vi "FT10_Fornax Energy Parameter Command.vi"(0 "Energy Channel ID":T4, 1 "Generator":T6="{\"Partition\":\"", 5 "Instrument Type":T5, 7 "Parameter Type":T3, 9 "Parameter Value":T2, 11 "Energy Mode":T1) -> (4 "JSON Command":string)   [LabVIEW 2015]
doc: "Build JSON command to adjust the mode or power on a specific port via Fornax. See Fornax manual > \"EnergyParameterCommand\" for more details."
uses:
  Controls/Control_Fornax Generator.ctl
  Controls/Control_Fornax Instrument Type.ctl
  Controls/Control_Fornax Energy Channel ID.ctl
  Controls/Control_Fornax Parameter Type.ctl
  Controls/Control_Fornax Parameter Value.ctl
  Controls/Control_Fornax Energy Mode.ctl
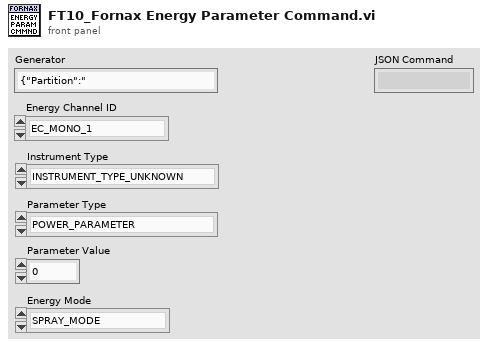
[diagram p1: front panel]
types:
  T1 = typedef "Control_Fornax Energy Mode.ctl" = enum16{"SPRAY_MODE", "CUT_MODE", "BLEND_MODE", "FULGERATE_MODE", "BIPOLAR_MODE", "VESSEL_SEALING_MODE", "VALLEYLAB_MODE", "BIPOLAR_RESECTION_CUT_MODE", "BIPOLAR_RESECTION_COAG_MODE", "AUTOBIPOLAR_MODE", "VIPER_HLA", "SOFT_COAG_MODE", "ECUT_MODE", "SHARED_SPRAY_MODE", "SHARED_FULGERATE_MODE", "CARDIO_MONO_MODE", "CARDIO_BIPOLAR_MODE", "BIPOLAR_LOW_MODE", "BIPOLAR_MACRO_MODE", "BIPOLAR_STANDARD_MODE", "BIPOLAR_MEDIUM_MODE", "VL_ENDOSCOPY_MODE", "NUM_ENERGY_MODES"}
  T2 = typedef "Control_Fornax Parameter Value.ctl" = i32
  T3 = typedef "Control_Fornax Parameter Type.ctl" = enum16{"POWER_PARAMETER", "CUT_MODALITY_POWER_PARAMETER", "COAG_MODALITY_POWER_PARAMETER", "VL_MODALITY_POWER_PARAMETER", "BY_MODE_POWER_PARAMETER", "VL_ENDO_CUT_MODALITY_POWER_PARAMETER", "VL_ENDO_COAG_MODALITY_POWER_PARAMETER", "VL_ENDO_COAG_ON_CUT_MODALITY_POWER_PARAMETER", "MODE_PARAMETER   (for changing Bipolar mode)", "CUT_MODALITY_MODE_PARAMETER  (for changing monopolar cut mode)", "COAG_MODALITY_MODE_PARAMETER (for changing monopolar coag mode)", "VL_ENDO_COAG_MODALITY_MODE_PARAMETER", "VL_ENDO_CUT_INTERVAL_PARAMETER", "VL_ENDO_CUT_DURATION_PARAMETER", "POWER_BAR_PARAMETER", "MAX_ACTIVATION_MSEC_TIME_PARAMETER", "AUTOBIPOLAR_DELAY_MSEC_TIME", "VL_ENDO_COAG_QUICK_ACCESS_PARAMETER"}
  T4 = typedef "Control_Fornax Energy Channel ID.ctl" = enum16{"EC_MONO_1  ", "EC_BIPOLAR  ", "EC_MONO_2  ", "EC_ADVANCED  ", "EC_ADVANCED_ECUT  ", "EC_ADVANCED_DCUT  ", "EC_SHARED_COAG  ", "EC_INTERNAL_BIP_CAL  "}
  T5 = typedef "Control_Fornax Instrument Type.ctl" = enum16{"INSTRUMENT_TYPE_UNKNOWN", "INSTRUMENT_TYPE_MONOPOLAR", "INSTRUMENT_TYPE_BIPOLAR", "INSTRUMENT_TYPE_TRIVERSE", "INSTRUMENT_TYPE_LIGASURE", "INSTRUMENT_TYPE_ADVANCE_II", "INSTRUMENT_TYPE_BIPOLAR_RESECTION", "INSTRUMENT_TYPE_HOOK", "INSTRUMENT_TYPE_BIZACT", "INSTRUMENT_TYPE_CARDIOBLATE_BIP", "INSTRUMENT_TYPE_CARDIOBLATE_BIP_GEMINI_S", "INSTRUMENT_TYPE_CARDIOBLATE_MONO", "INSTRUMENT_TYPE_ULTRASONIC", "INSTRUMENT_TYPE_MONOPOLAR_GI ", "INSTRUMENT_TYPE_GOLDILOCKS "}
  T6 = typedef "Control_Fornax Generator.ctl" = string
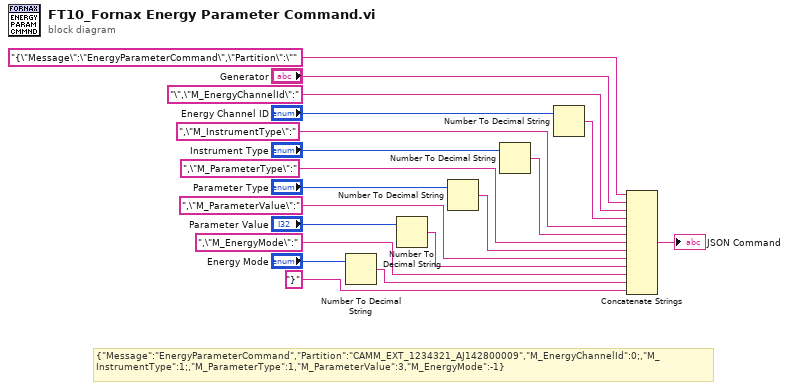
[diagram p0: block diagram]
diagram:
  # "{\"Message\":\"EnergyParameterCommand\",\"Partition\":\"CAMM_EXT_1234321_AJ142800009\",\"M_EnergyChannelId\":0;,\"M_InstrumentType\":1;,\"M_ParameterType\":1,\"M_ParameterValue\":3,\"M_EnergyMode\":-1}"
  n1 = Number To Decimal String(number="Energy Mode") -> (decimal integer string=w2:string)  [unwired: 1 in]
  n2 = Number To Decimal String(number="Parameter Value") -> (decimal integer string=w4:string)  [unwired: 1 in]
  n3 = Number To Decimal String(number="Parameter Type") -> (decimal integer string=w8:string)  [unwired: 1 in]
  n4 = Number To Decimal String(number="Instrument Type") -> (decimal integer string=w10:string)  [unwired: 1 in]
  n5 = Number To Decimal String(number="Energy Channel ID") -> (decimal integer string=w12:string)  [unwired: 1 in]
  n6 = Concatenate Strings("{\"Message\":\"EnergyParameterCommand\",\"Partition\":\"", "Generator", "\",\"M_EnergyChannelId\":", w12, ",\"M_InstrumentType\":", w10, ",\"M_ParameterType\":", w8, ",\"M_ParameterValue\":", w4, ",\"M_EnergyMode\":", w2, "}") -> (→"JSON Command":string)
